vi "Remove Invisible Characters from String.vi"(1 "Remove Line Feed. etc (F)":bool, 3 "String":string) -> (0 "result string":string)   [LabVIEW 2021, in "Strings.lvlib"]
doc: "Removes <B>space</B> and <B>TAB</B> characters from a string.\n\nOptionally, also removes all end of line characters."
uses:
  Strings.lvlib
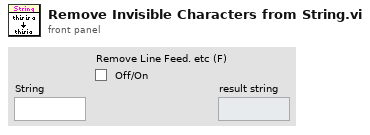
[diagram p1: front panel]
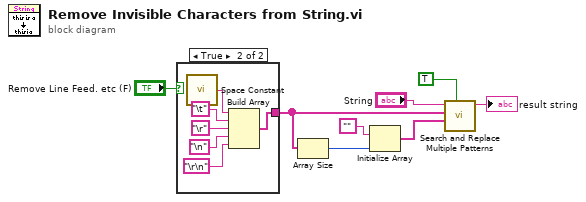
[diagram p0: block diagram]
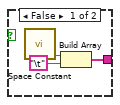
[diagram p2: hidden frame]
diagram:
  n1 = case shown="True" "Remove Line Feed. etc (F)" {
    tunnel: [w9 w15] -> w4
    frame False {
      n2 = call <vilib>:"Space Constant.vi"() -> ("String"=w11:string)
      n3 = Build Array(w11, "\t") -> (w9:string[])
    }
    frame True {
      n4 = call <vilib>:"Space Constant.vi"() -> ("String"=w17:string)
      n5 = Build Array(w17, "\t", "\r", "\n", "\r\n") -> (w15:string[])
    }
  }
  n6 = Array Size(array=w4) -> (size(s)=w3:i32)
  n7 = Initialize Array("", w3) -> (w1:string[])
  n8 = call "Search and Replace Multiple Patterns.vi"("replace all? (F)"=TRUE, "replace strings (\"\")"=w1, "regular expressions"=w4, "source"="String") -> ("result string"=→"result string":string)  [unwired: 6 in, 1 out]
